vi "JSON - Decode JSON String into Cluster.vi"(8 "error in":errorcluster, 11 "JSON String":string="{\n\r \"timestamp\":4169579306,\n\r \"adc\":[\n\r  {\"time\":0, \"ch\":0, \"data\":0},\n\r  {\"time\":0, \"ch\":1, \"data\":12},\n\r ],\n\r}") -> (0 "error out":errorcluster, 2 "Data out":T1)   [LabVIEW 2021]
doc: "Decode a JSON string into a cluster (typedef)"
uses:
  TypeDefs/TypeDef - Cluster Representing Decoded JSON Message.ctl
  <vilib>/addons/_JKI.lib/Serialization/JSON/JKI JSON Serialization.lvlib
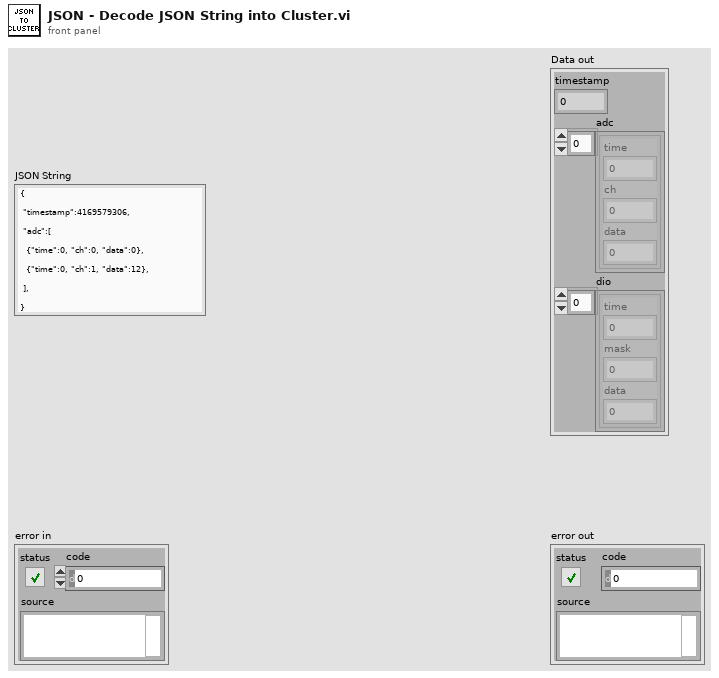
[diagram p1: front panel]
types:
  T1 = typedef "TypeDef - Cluster Representing Decoded JSON Message.ctl" = cluster{"timestamp":u64, "adc":cluster{"time":i32, "ch":i32, "data":i32}[], "dio":cluster{"time":i32, "mask":i32, "data":u16}[]}
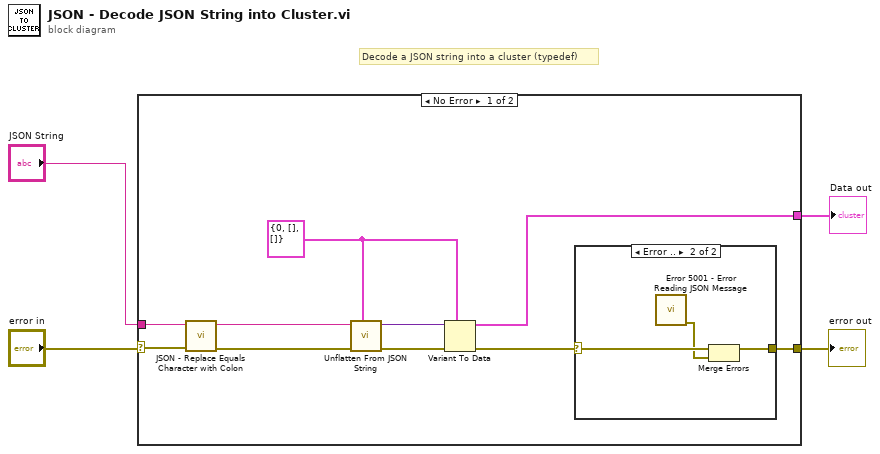
[diagram p0: block diagram]
diagram:
  # "Decode a JSON string into a cluster (typedef)"
  n1 = case shown="No Error" "error in" {
    selector: "error in" -> [w5 w19]
    tunnel: "JSON String" -> [w13 _]
    tunnel: [w8 _] -> w3
    tunnel: [w6 w19] -> w2
    frame No Error {
      w12 = T1 {"timestamp"=0, "adc"=[], "dio"=[]}
      n2 = call "JSON - Replace Equals Character with Colon.vi"("error in"=w5, "Input JSON String"=w13) -> ("error out"=w11:errorcluster, "Output JSON String"=w9:string)  [unwired: 8 in]
      n3 = call <vilib>:"Unflatten From JSON String.vi"("Type and Defaults"=w12, "error in"=w11, "JSON String"=w9) -> ("error out"=w10:errorcluster, "Variant"=w14:variant)  [unwired: 7 in]
      n4 = Variant To Data(error in=w10, type=w12, Variant=w14) -> (data=w8:T1, error out=w7:errorcluster)
      n5 = case shown="Error .." w7 {
        selector: w7 -> [w15 w17]
        tunnel: [w15 w18] -> w6
        frame No Error {
        }
        frame Error {
          n6 = call "Error 5001 - Error Reading JSON Message.vi"() -> ("error out"=w16:errorcluster)  [unwired: 11 in]
          n7 = Merge Errors(w17, w16) -> (w18:errorcluster)
        }
      }
    }
    frame Error {
    }
  }
  "error out" <- w2
  "Data out" <- w3
